vi "Style List To Object.vi"(3 "Style List":T1) -> (1 "Style Object":refnum<class "Style.lvclass">)   [LabVIEW 2017, in "Styles.lvlib"]
uses:
  Styles.lvlib
  Style List--enum.ctl
  Style/Style.lvclass
  Title/Title.lvclass
  C:/Users/Neo/Desktop/Dev_Tools_BR/LabVIEW_NPOI/src/Styles/Style/Style.lvclass
  Heading 1/Heading 1.lvclass
  Heading 2/Heading 2.lvclass
  Heading 3/Heading 3.lvclass
  Figure/Figure.lvclass
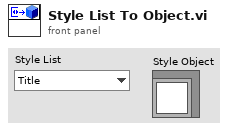
[diagram p1: front panel]
types:
  T1 = typedef "Styles.lvlib/Style List--enum.ctl" = enum16{"Title", "Heading 1", "Heading 2", "Heading 3", "Normal", "Figure"}
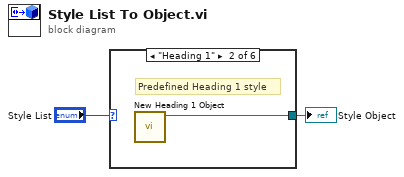
[diagram p0: block diagram]
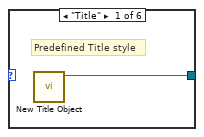
[diagram p2: hidden frame]
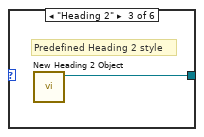
[diagram p3: hidden frame]
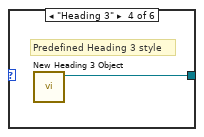
[diagram p4: hidden frame]
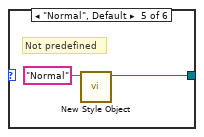
[diagram p5: hidden frame]
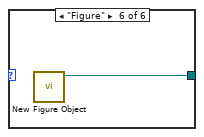
[diagram p6: hidden frame]
diagram:
  n1 = case shown="\"Heading 1\"" "Style List" {
    tunnel: [w3 w4 w5 w6 w8 w9] -> w1
    frame "Title" {
      # "Predefined Title style"
      n2 = call "New Title Object.vi"() -> ("Title out"=w3:refnum<class "Title.lvclass">)  [unwired: 10 in, 1 out]
    }
    frame "Heading 1" {
      # "Predefined Heading 1 style"
      n3 = call "New Heading 1 Object.vi"() -> ("Heading 1 out"=w4:refnum<class "Heading 1.lvclass">)  [unwired: 10 in, 1 out]
    }
    frame "Heading 2" {
      # "Predefined Heading 2 style"
      n4 = call "New Heading 2 Object.vi"() -> ("Heading 2 out"=w5:refnum<class "Heading 2.lvclass">)  [unwired: 10 in, 1 out]
    }
    frame "Heading 3" {
      # "Predefined Heading 3 style"
      n5 = call "New Heading 3 Object.vi"() -> ("Heading 3 out"=w6:refnum<class "Heading 3.lvclass">)  [unwired: 10 in, 1 out]
    }
    frame "Normal", Default {
      # "Not predefined"
      # "Not predefined"
      n6 = call "New Style Object.vi"("Style Name"="Normal") -> ("Style out"=w8:refnum<class "Style.lvclass">)  [unwired: 9 in, 1 out]
    }
    frame "Figure" {
      n7 = call "New Figure Object.vi"() -> ("Figure out"=w9:refnum<class "Figure.lvclass">)  [unwired: 10 in, 1 out]
    }
  }
  "Style Object" <- w1
